vi "RunCore.vi"(8 "Error In":errorcluster, 9 "Timeout (s)":dbl, 10 "MeasIn":refnum<class "IAction.lvclass">, 11 "HardwareIn":refnum<class "IReference.lvclass">) -> (0 "Error Out":errorcluster, 1 "Timeout?":bool, 2 "ResultOut":refnum<class "IResult.lvclass">, 3 "HardwareOut":refnum<class "IReference.lvclass">)   [LabVIEW 2019, in "IAction.lvclass"]
uses:
  IAction.lvclass
  IReference/IReference.lvclass
  IResult/IResult.lvclass
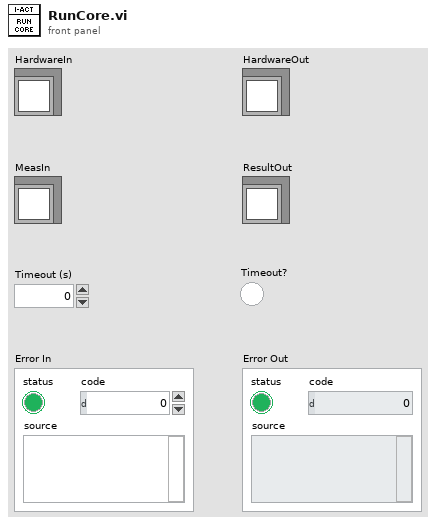
[diagram p1: front panel]
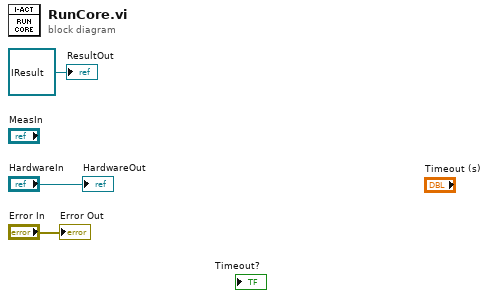
[diagram p0: block diagram]
diagram:
  "Error Out" <- "Error In"
  "HardwareOut" <- "HardwareIn"
  "ResultOut" <- refnum<class "IResult.lvclass"> refnum ("IResult.lvclass")
